vi "LayoutFGV.vi"(7 "String":string, 8 "Variant":variant, 9 "name":string, 10 "file (use dialog)":path, 11 "InitRef":T1) -> ()   [LabVIEW 2020, in "MDI ViewManager.lvlib"]
uses:
  MDI ViewManager.lvlib
  <vilib>/Utility/miscctls.llb/LVPointTypeDef.ctl
  <vilib>/Utility/miscctls.llb/LVBoundsTypeDef.ctl
  <vilib>/Utility/miscctls.llb/LVPositionTypeDef.ctl
  Typedef/UpdateInsertableVICtl.ctl
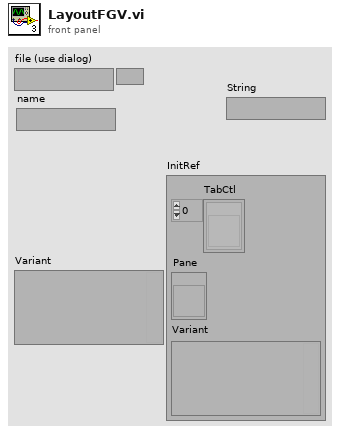
[diagram p1: front panel]
types:
  T1 = cluster{"TabCtl":refnum<vi>[], "Pane":refnum<vi>, "Variant":variant}
  T2 = typedef "LVPointTypeDef.ctl" = cluster{"Horizontal":i16, "Vertical":i16}
  T3 = typedef "LVBoundsTypeDef.ctl" = cluster{"Width":u32, "Height":u32}
  T4 = typedef "LVPositionTypeDef.ctl" = cluster{"Left":i32, "Top":i32}
  T5 = cluster{"Origin":T2, "Layout":cluster{"Pane Dimension":T3, "Position":T4, "Label":string, "Visible":bool, "InsertedViewName":string}[]}
  T6 = typedef "MDI ViewManager.lvlib/UpdateInsertableVICtl.ctl" = cluster{"Name":string, "VIPath":path, "Height(Default)":dbl, "Widht(Default)":dbl}
  T7 = cluster{"Pane Dimension":T3, "Position":T4, "Label":string, "Visible":bool, "InsertedViewName":string}
  T8 = cluster{"Pane Dimension":T3, "Position":T4, "Label":string, "Visible":bool, "InsertedViewName":string}[]
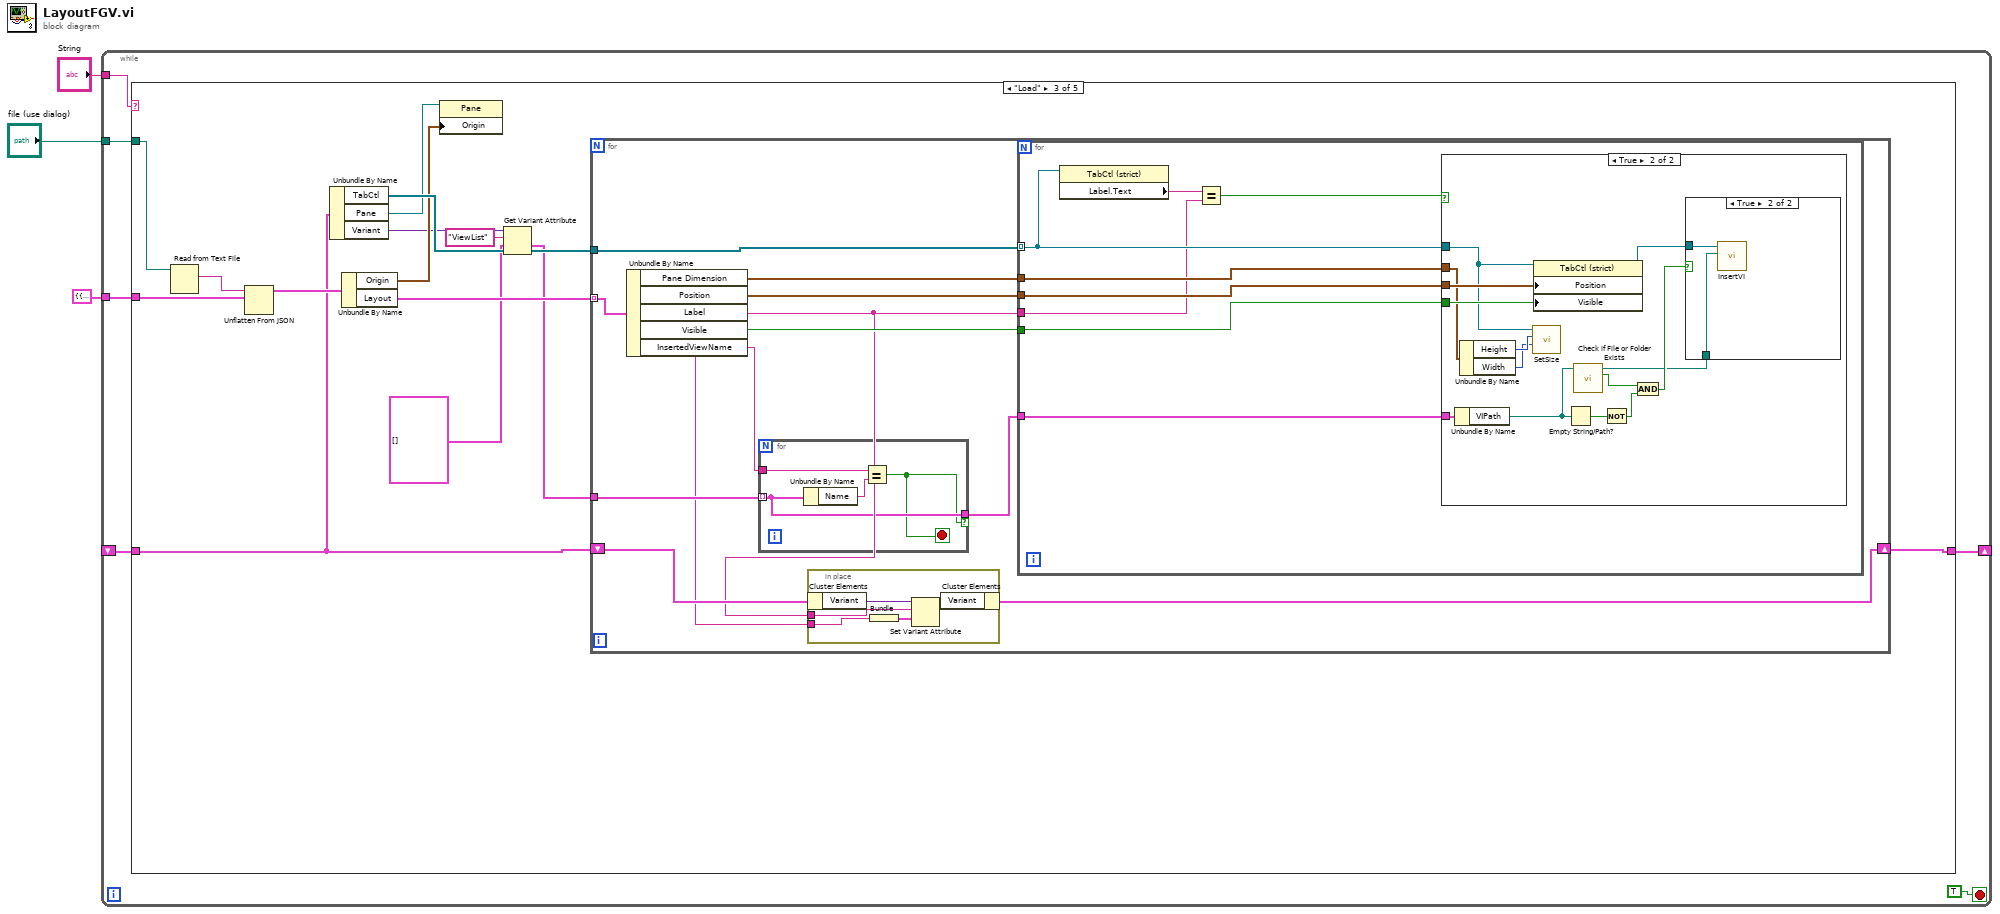
[diagram p0: block diagram]
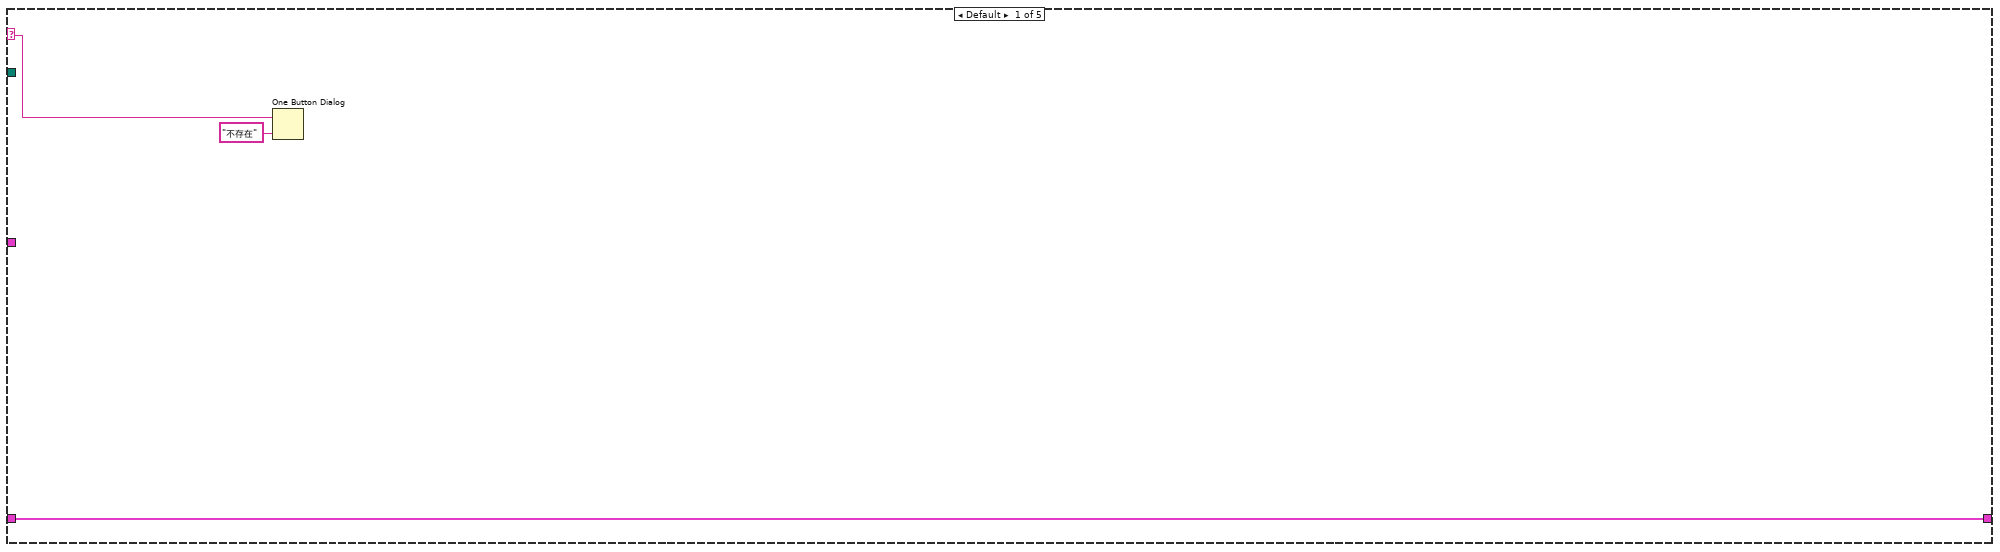
[diagram p2: hidden frame]
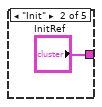
[diagram p3: hidden frame]
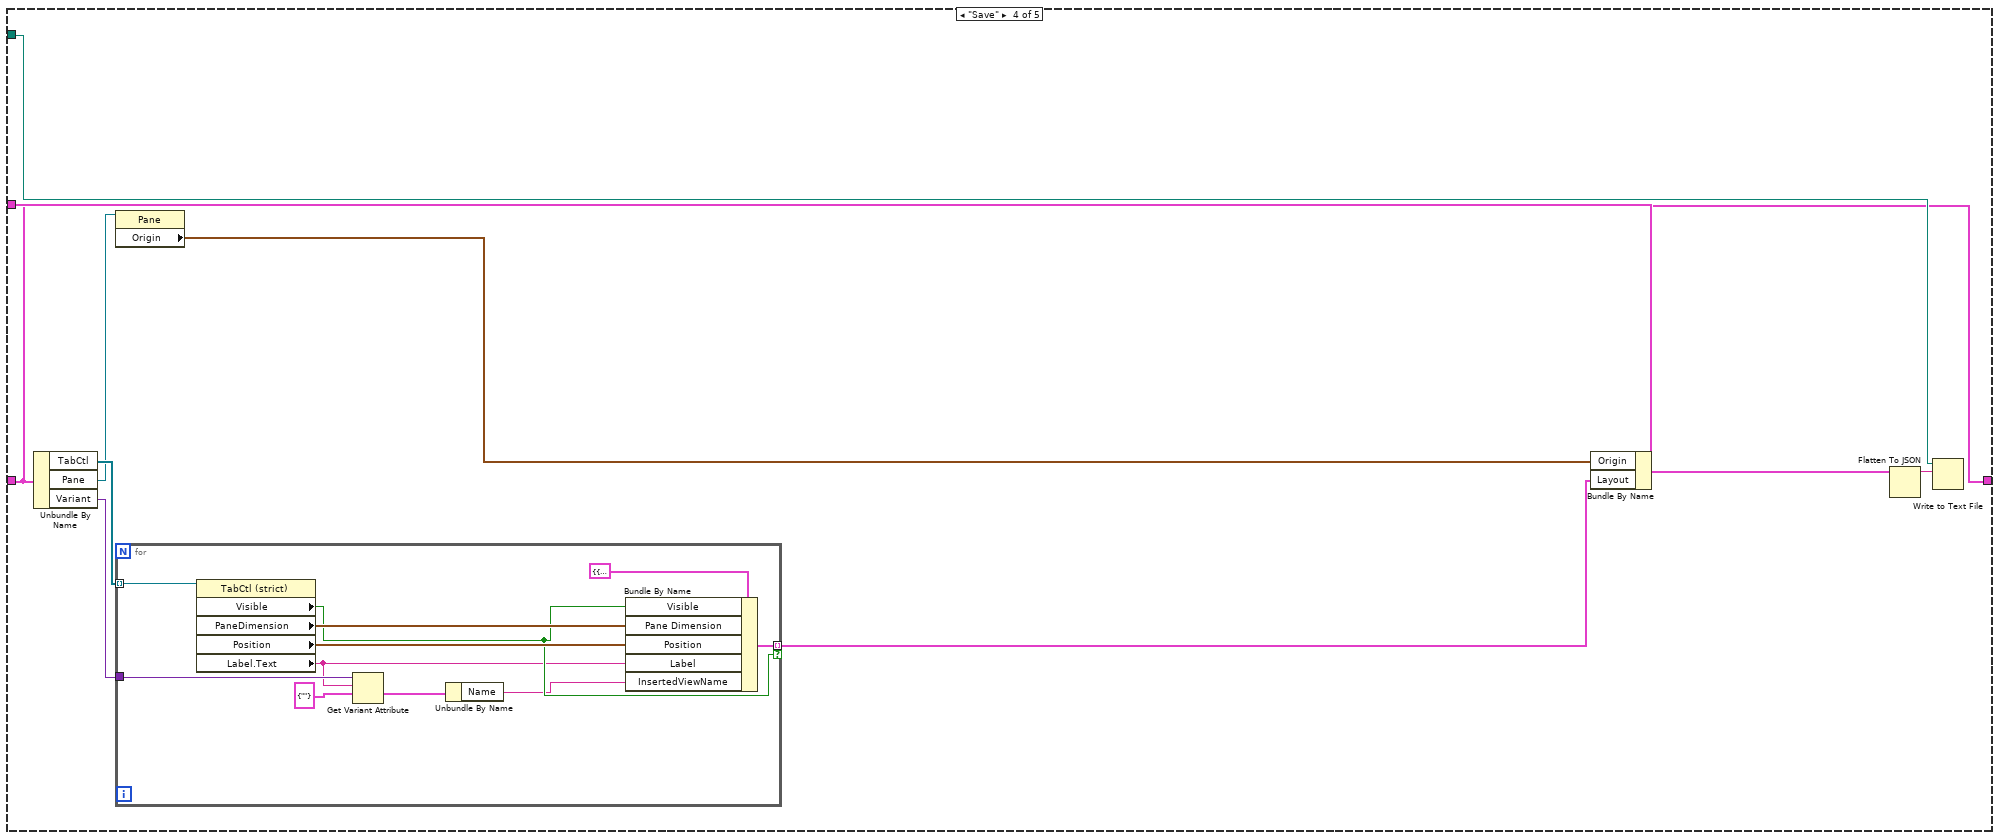
[diagram p6: hidden frame]
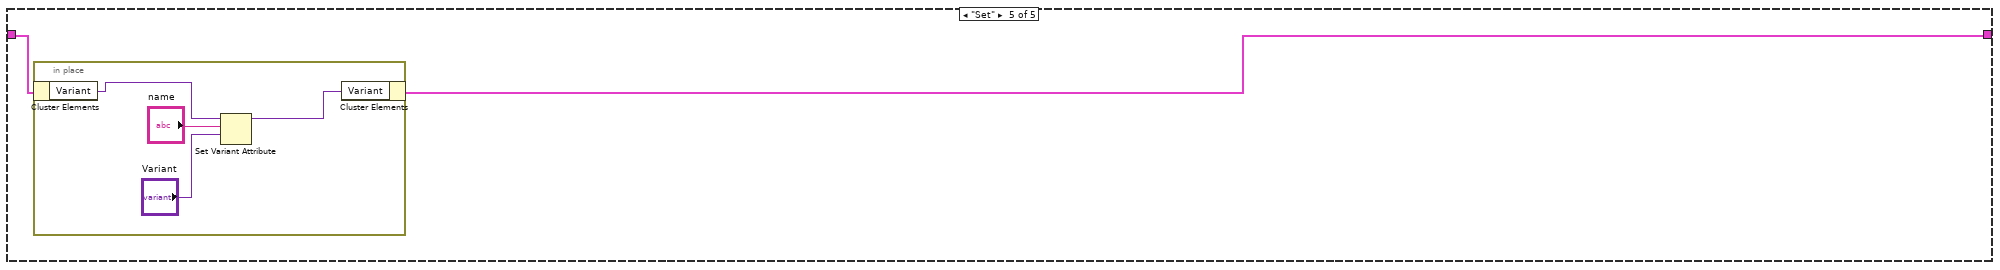
[diagram p7: hidden frame]
diagram:
  n1 = while {
    tunnel: "String" -> [w7]
    tunnel: "file (use dialog)" -> [w6]
    shift-right: [w5] -> _
    shift-left: _ -> [w8]
    tunnel: T5 {"Origin"={"Horizontal"=0, "Vertical"=0}, "Layout"=[]} -> [w4]
    stop <- TRUE stop-if-true
    n2 = case shown="\"Load\"" w7 {
      selector: w7 -> [w11 _ _ _ _]
      tunnel: w8 -> [w12 _ w15 w75 w94]
      tunnel: w6 -> [_ _ w26 w80 _]
      tunnel: [w12 "InitRef" w14 w75 w93] -> w5
      tunnel: w4 -> [_ _ w25 w76 _]
      frame Default {
        n3 = One Button Dialog(message=w11, button name ("OK")="不存在") -> ()  [unwired: 1 out]
      }
      frame "Init" {
      }
      frame "Load" {
        n4 = Read from Text File(file (use dialog)=w26) -> (text=w27:string)  [unwired: 3 in, 3 out]
        n5 = Unflatten From JSON(JSON string=w27, type and defaults=w25) -> (value=w24:T5)  [unwired: 5 in, 1 out]
        n6 = Unbundle By Name(w15) -> ("TabCtl"=w22:refnum<vi>[], "Pane"=w21:refnum<vi>, "Variant"=w19:variant)
        n7 = Unbundle By Name(w24) -> ("Origin"=w20:T2, "Layout"=w23:T8)
        n8 = property class="Pane"(reference=w21, "Origin"=w20) -> ()  [unwired: 1 in, 2 out]
        n9 = Get Variant Attribute(Variant=w19, name="ViewList", default value (empty Variant)=T6[] [] ("1.Val.UpdateInsertableVI")) -> (value=w16:T6[])  [unwired: 1 in, 3 out]
        n10 = for {
          tunnel: w23 -> [w37] mode=indexing
          tunnel: w22 -> [w38]
          tunnel: w16 -> [w33]
          shift-right: [w30] -> w14
          shift-left: w15 -> [w31]
          n11 = Unbundle By Name(w37) -> ("Pane Dimension"=w36:T3, "Position"=w35:T4, "Label"=w29:string, "Visible"=w34:bool, "InsertedViewName"=w28:string)
          n12 = for {
            tunnel: w33 -> [w47] mode=indexing
            tunnel: [w47] -> w32 if=w46
            tunnel: w28 -> [w45]
            stop <- w46 stop-if-true
            n13 = Unbundle By Name(w47) -> ("Name"=w44:string)
            n14 = Equal?(x=w45, y=w44) -> (x = y?=w46:bool)
          }
          n15 = in-place {
            in-place-border: w29 -> [w41]
            in-place-border: w28 -> [w40]
            n16 = in-place-cluster #1(w31) -> ("Variant"=w43:variant)
            n17 = Bundle("InsertedViewName"=w40) -> (w39:cluster{"InsertedViewName":string})  [unwired: 1 in]
            n18 = Set Variant Attribute(Variant=w43, name=w41, value=w39) -> (Variant out=w42:variant)  [unwired: 1 in, 2 out]
            n19 = in-place-cluster #1("Variant"=w42) -> (w30:T1)
          }
          n20 = for {
            tunnel: w38 -> [w55] mode=indexing
            tunnel: w36 -> [w52]
            tunnel: w35 -> [w51]
            tunnel: w29 -> [w50]
            tunnel: w34 -> [w49]
            tunnel: w32 -> [w48]
            n21 = property class="TabCtl (strict)"(reference=w55) -> ("Label.Text"=w54:string)  [unwired: 1 in, 2 out]
            n22 = Equal?(x=w54, y=w50) -> (x = y?=w53:bool)
            n23 = case shown="True" w53 {
              tunnel: w52 -> [_ w58]
              tunnel: w51 -> [_ w69]
              tunnel: w49 -> [_ w68]
              tunnel: w55 -> [_ w59]
              tunnel: w48 -> [_ w66]
              frame False {
              }
              frame True {
                n24 = Unbundle By Name(w66) -> ("VIPath"=w65:path)
                n25 = Unbundle By Name(w58) -> ("Height"=w57:u32, "Width"=w56:u32)
                n26 = call "SetSize.vi"("Widht"=w56, "Height"=w57, "TabControl in"=w59) -> ()  [unwired: 7 in, 2 out]
                n27 = property class="TabCtl (strict)"(reference=w59, "Position"=w69, "Visible"=w68) -> (reference out=w67:refnum<vi>)  [unwired: 1 in, 1 out]
                n28 = Empty String/Path?(string/path=w65) -> (empty?=w63:bool)
                n29 = call <vilib>:"Check if File or Folder Exists.vi"("path"=w65) -> ("file or folder exists?"=w64:bool, "dup path"=w60:path)  [unwired: 8 in, 1 out]
                n30 = Not(x=w63) -> (.not. x?=w62:bool)
                n31 = And(x=w64, y=w62) -> (x .and. y?=w61:bool)
                n32 = case shown="True" w61 {
                  tunnel: w67 -> [_ w71]
                  tunnel: w60 -> [_ w70]
                  frame False {
                  }
                  frame True {
                    n33 = call "InsertVI.vi"("VIPath"=w70, "TabControl in"=w71) -> ()  [unwired: 8 in, 2 out]
                  }
                }
              }
            }
          }
        }
      }
      frame "Save" {
        n34 = Unbundle By Name(w75) -> ("TabCtl"=w74:refnum<vi>[], "Pane"=w73:refnum<vi>, "Variant"=w72:variant)
        n35 = property class="Pane"(reference=w73) -> ("Origin"=w79:T2)  [unwired: 1 in, 2 out]
        n36 = for {
          tunnel: w74 -> [w87] mode=indexing
          tunnel: [w90] -> w78 mode=indexing if=w88
          tunnel: w72 -> [w86]
          n37 = property class="TabCtl (strict)"(reference=w87) -> ("Visible"=w88:bool, "PaneDimension"=w92:T3, "Position"=w91:T4, "Label.Text"=w85:string)  [unwired: 1 in, 2 out]
          n38 = Get Variant Attribute(Variant=w86, name=w85, default value (empty Variant)=cluster{"Name":string} {"Name"=""} ("output cluster")) -> (value=w83:cluster{"Name":string})  [unwired: 1 in, 3 out]
          n39 = Unbundle By Name(w83) -> ("Name"=w82:string)
          n40 = Bundle By Name(cluster=T7 {"Pane Dimension"={"Width"=0, "Height"=0}, "Position"={"Left"=0, "Top"=0}, "Label"="", "Visible"=FALSE, "InsertedViewName"=""}, "Visible"=w88, "Pane Dimension"=w92, "Position"=w91, "Label"=w85, "InsertedViewName"=w82) -> (w90:T7)
        }
        n41 = Bundle By Name(cluster=w76, "Origin"=w79, "Layout"=w78) -> (w77:T5)
        n42 = Flatten To JSON(anything=w77) -> (JSON string=w81:string)  [unwired: 2 in, 1 out]
        n43 = Write to Text File(file (use dialog)=w80, text=w81) -> ()  [unwired: 2 in, 3 out]
      }
      frame "Set" {
        n44 = in-place {
          n45 = in-place-cluster #2(w94) -> ("Variant"=w98:variant)
          n46 = Set Variant Attribute(Variant=w98, name="name", value="Variant") -> (Variant out=w97:variant)  [unwired: 1 in, 2 out]
          n47 = in-place-cluster #2("Variant"=w97) -> (w93:T1)
        }
      }
    }
  }
